vi "MGI CheckValue Directory Compare.vi"(5 "U32 Slider Ref (Use Progress Bar Dialog)":refnum<vi>, 7 "CheckValue Type (Checksum)":T1, 8 "error in (no error)":errorcluster, 9 "Expected CheckValue U32[i]":u32[](array[numeric]) format="%.0x", 10 "Relative Path[i]":path[](array[path]), 11 "Path":path) -> (0 "error out":errorcluster, 1 "Missing?[i]":bool[](array[boolean]), 2 "Missmatch or Missing?[i]":bool[](array[boolean]), 3 "All Match?":bool, 4 "Aborted?":bool, 6 "Actual CheckValue U32[i]":u32[](array[numeric]) format="%.0x")   [LabVIEW 2020]
doc: "Compare the specified expected files and checkvalues to the specified directory. Extra files in the directory are ignored. If all expected files match, then output true, otherwise output false.\nIf a reference to a slider is wired, then the slider is updated to show the progress of the comparison. Otherwise show a progress bar dialog with optional abort button.\n\nAuthored by Shawn Walpole\nsupport@mooregoodideas.com\nwww.mooregoodideas.com\n\nCopyright (c) 2010, Moore Good Ideas, Inc.\n\nAll rights reserved.\n\nRedistribution and use in source and binary forms, with or without modification, are permitted provided that the following conditions are met:\n\n * Redistributions of source code must retain the above copyright notice, this list of conditions and the following disclaimer.\n * Redistributions in binary form must reproduce the above copyright notice, this list of conditions and the following disclaimer in the documentation and/or other materials provided with the distribution.\n * Neither the name of Moore Good Ideas, Inc. nor the names of its contributors may be used to endorse or promote products derived from this software without specific prior written permission.\n\nTHIS SOFTWARE IS PROVIDED BY THE COPYRIGHT HOLDERS AND CONTRIBUTORS \"AS IS\" AND ANY EXPRESS OR IMPLIED WARRANTIES, INCLUDING, BUT NOT LIMITED TO, THE IMPLIED WARRANTIES OF MERCHANTABILITY AND FITNESS FOR A PARTICULAR PURPOSE ARE DISCLAIMED. IN NO EVENT SHALL THE COPYRIGHT OWNER OR CONTRIBUTORS BE LIABLE FOR ANY DIRECT, INDIRECT, INCIDENTAL, SPECIAL, EXEMPLARY, OR CONSEQUENTIAL DAMAGES (INCLUDING, BUT NOT LIMITED TO, PROCUREMENT OF SUBSTITUTE GOODS OR SERVICES; LOSS OF USE, DATA, OR PROFITS; OR BUSINESS INTERRUPTION) HOWEVER CAUSED AND ON ANY THEORY OF LIABILITY, WHETHER IN CONTRACT, STRICT LIABILITY, OR TORT (INCLUDING NEGLIGENCE OR OTHERWISE) ARISING IN ANY WAY OUT OF THE USE OF THIS SOFTWARE, EVEN IF ADVISED OF THE POSSIBILITY OF SUCH DAMAGE."
uses:
  <userlib>/_MGI/File/Checksum/MGI CheckValue Method Enum.ctl
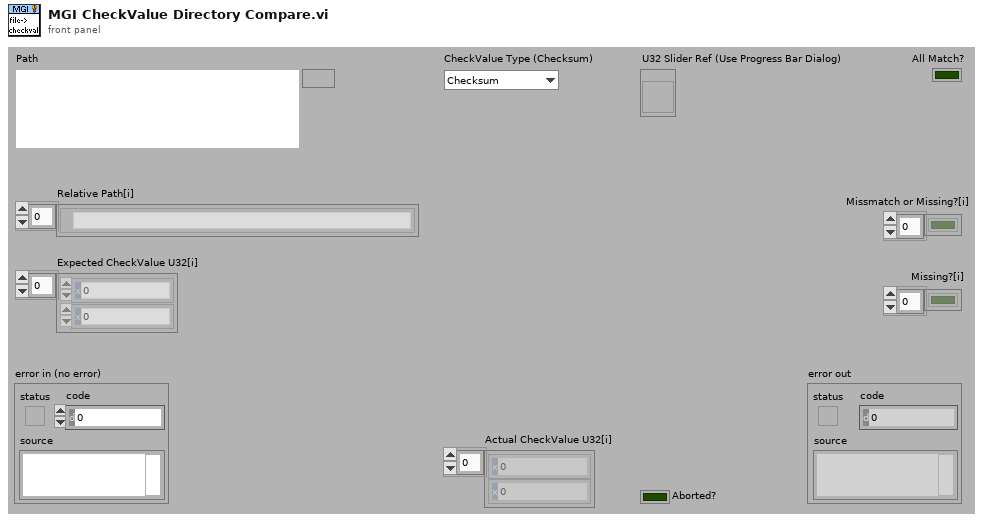
[diagram p1: front panel]
types:
  T1 = typedef "MGI CheckValue Method Enum.ctl" = enum16{"Checksum", "XOr"}
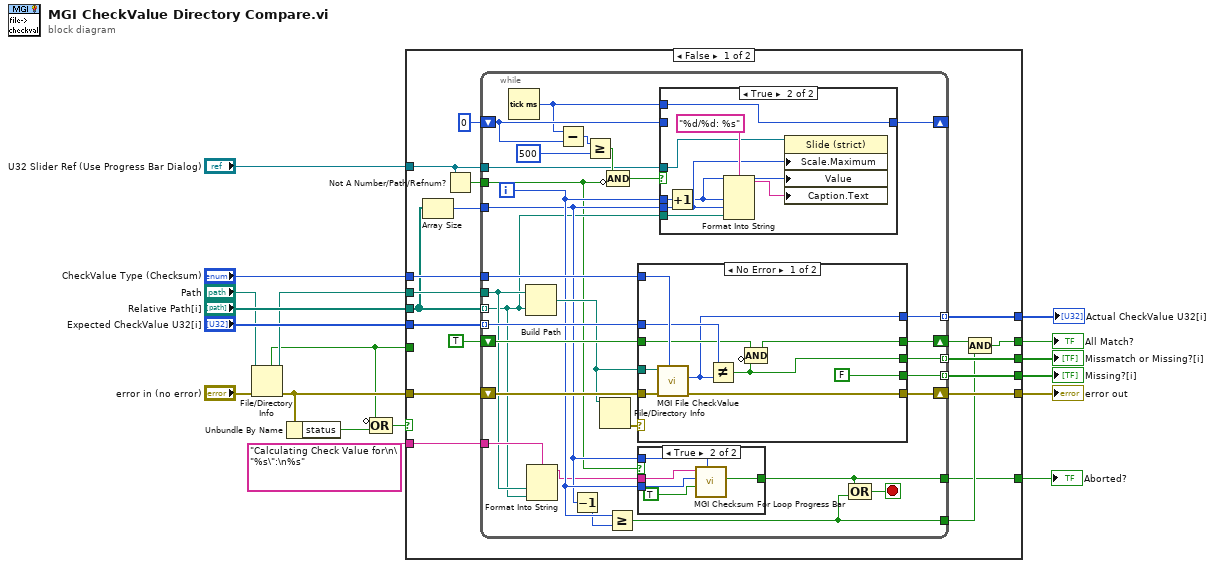
[diagram p0: block diagram]
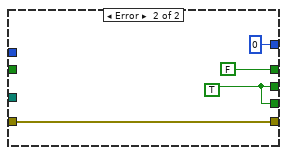
[diagram p4: hidden frame]
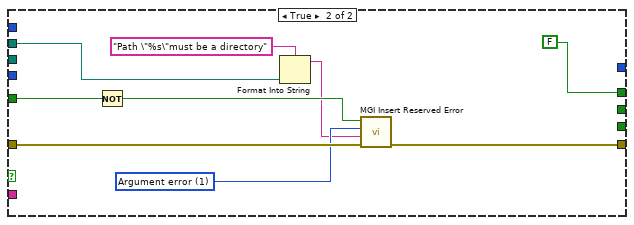
[diagram p5: hidden frame]
diagram:
  n1 = File/Directory Info(path="Path", error in="error in (no error)") -> (path out=w12:path, directory=w7:bool, error out=w9:errorcluster)  [unwired: 4 out]
  n2 = Unbundle By Name(w9) -> ("status"=w11:bool)
  n3 = Compound Arithmetic op=OR(invert w7, w11) -> (w10:bool)
  n4 = case shown="False" w10 {
    tunnel: "Relative Path[i]" -> [w24 _]
    tunnel: "Expected CheckValue U32[i]" -> [w37 _]
    tunnel: "CheckValue Type (Checksum)" -> [w36 _]
    tunnel: [w25 FALSE] -> w15
    tunnel: w12 -> [w34 w98]
    tunnel: w9 -> [w33 w104]
    tunnel: [w32 w103] -> w8
    tunnel: w7 -> [_ w101]
    tunnel: [w31 _] -> w6
    tunnel: [w30 _] -> w5
    tunnel: "U32 Slider Ref (Use Progress Bar Dialog)" -> [w27 _]
    tunnel: "Calculating Check Value for\n\"%s\":\n%s" ("format string") -> [w21 _]
    tunnel: [w20 _] -> w2
    tunnel: [w19 _] -> w1
    frame False {
      n5 = Array Size(array=w24) -> (size(s)=w23:i32)
      n6 = Not A Number/Path/Refnum?(number/path/refnum=w27) -> (NaN/Path/Refnum?=w29:bool)
      n7 = while {
        tunnel: w24 -> [w44] mode=indexing
        tunnel: w37 -> [w65] mode=indexing
        tunnel: w34 -> [w45]
        shift-right: [w58] -> w32
        shift-left: w33 -> [w67]
        tunnel: w36 -> [w66]
        shift-right: [w63] -> w26
        shift-left: TRUE -> [w64]
        tunnel: [w62] -> w31 mode=indexing
        tunnel: [w59] -> w30 mode=indexing
        shift-right: [w51] -> _
        shift-left: u32 0 ("millisecond timer value") -> [w52]
        tunnel: w27 -> [w53]
        tunnel: w29 -> [w40]
        tunnel: w23 -> [w48]
        tunnel: [w42] -> w22
        tunnel: w21 -> [w46]
        tunnel: [w39] -> w20
        tunnel: [w38] -> w19 mode=indexing
        i -> [w49]
        stop <- w41 stop-if-true
        n8 = Tick Count (ms)() -> (millisecond timer value=w50:u32)
        n9 = Build Path(base path=w45, name or relative path=w44) -> (appended path=w61:path)
        n10 = Format Into String(format string=w46, w45, w44) -> (resulting string=w43:string)  [unwired: 2 in, 1 out]
        n11 = Subtract(x=w50, y=w52) -> (x-y=w57:u32)
        n12 = Decrement(x=w48) -> (x-1=w47:i32)
        n13 = Greater Or Equal?(x=w57, y=u32 500) -> (x >= y?=w56:bool)
        n14 = File/Directory Info(path=w61) -> (error out=w60:errorcluster)  [unwired: 1 in, 6 out]
        n15 = Compound Arithmetic op=AND(w56, invert w40) -> (w54:bool)
        n16 = Greater Or Equal?(x=w49, y=w47) -> (x >= y?=w42:bool)
        n17 = case shown="No Error" w60 {
          tunnel: w67 -> [w91 w95]
          tunnel: w66 -> [w90 _]
          tunnel: w65 -> [w89 _]
          tunnel: w64 -> [w88 _]
          tunnel: [w87 FALSE] -> w63
          tunnel: [w84 w94] -> w62
          tunnel: w61 -> [w86 _]
          tunnel: [FALSE w94] -> w59
          tunnel: [w83 w95] -> w58
          tunnel: [w82 u32 0 ("CheckValue")] -> w38
          frame No Error {
            n18 = call <userlib>:"MGI File CheckValue.vi"("CheckValue Type"=w90, "error in (no error)"=w91, "File"=w86) -> ("error out"=w83:errorcluster, "CheckSum"=w82:u32)  [unwired: 7 in]
            n19 = Not Equal?(x=w89, y=w82) -> (x != y?=w84:bool)
            n20 = Compound Arithmetic op=AND(w88, invert w84) -> (w87:bool)
          }
          frame Error {
            w94 = TRUE
          }
        }
        n21 = case shown="True" w40 {
          tunnel: w49 -> [_ w70]
          tunnel: w48 -> [_ w68]
          tunnel: w43 -> [_ w71]
          tunnel: [_ w72] -> w39
          frame False {
          }
          frame True {
            n22 = call <userlib>:"MGI Checksum For Loop Progress Bar.vi"("Total Iter"=w68, "Allow Abort?(F)"=TRUE, "Current Iter"=w70, "Message"=w71) -> ("Aborted?"=w72:bool)  [unwired: 6 in, 1 out]
          }
        }
        n23 = case shown="True" w54 {
          tunnel: w53 -> [_ w78]
          tunnel: w49 -> [_ w75]
          tunnel: w48 -> [_ w79]
          tunnel: w52 -> [w73 _]
          tunnel: [w73 w77] -> w51
          tunnel: w50 -> [_ w77]
          tunnel: w44 -> [_ w76]
          frame False {
          }
          frame True {
            n24 = Increment(x=w75) -> (x+1=w74:i32)
            n25 = Format Into String(format string="%d/%d: %s", w74, w79, w76) -> (resulting string=w81:string)  [unwired: 2 in, 1 out]
            n26 = property class="Slide (strict)"(reference=w78, "Scale.Maximum"=w79, "Value"=w74, "Caption.Text"=w81) -> ()  [unwired: 1 in, 2 out]
          }
        }
        n27 = Compound Arithmetic op=OR(w39, w42) -> (w41:bool)
      }
      n28 = Compound Arithmetic op=AND(w26, w22) -> (w25:bool)
    }
    frame True {
      w99 = u16 1 items=["No error", "Argument error", "Memory is full", "Out of zone", "End of file", "File already open", "Generic file I/O error", "File not found", "File permission error", "Disk is full", "Duplicate path", "Too many files open", "System feature not enabled", "Resource file not found", "Cannot add resource", "Resource not found", "Image not found", "Image memory error", "Pen does not exist", "Config type invalid", "Config token not found", "Config parse error", "Config memory error", "Bad external code format", "Bad external code offset", "External code not present", "Null window", "Destroy window error", "Null menu", "Print aborted", "Bad print record", "Print driver error", "Windows error during printing", "Memory error during printing", "Print dialog error", "Generic print error", "Invalid device refnum", "Device not found", "Device parameter error", "Device unit error", "Cannot open device", "Device call aborted", "Generic error", "Cancelled by user", "Object ID too low", "Object ID too high", "Object not in heap", "Unknown heap", "Unknown object (invalid DefProc)", "Unknown object (DefProc not in table)", "Message out of range", "Invalid (null) method", "Unknown message", "Manager call not supported", "Bad address", "Network operation in progress", "Network operation timed out", "Connection is busy", "Network attribute not supported", "Network error", "Address in use", "System out of memory", "Connection aborted", "Connection refused", "Not connected", "Already connected", "Connection closed", "Initialization error (interapplication manager)", "Bad occurrence", "Wait on unbound occurrence handler", "Occurrence queue overflow", "Datalog type conflict", "Unused", "Unrecognized type (interapplication manager)", "Memory corrupt", "Failed to make temporary DLL", "Old CIN version", "Drag socket not found", "Failed to load drop-object", "Failed to register OLE object", "Failed to release OLE object", "Format specifier type mismatch", "Unknown format specifier", "Too few format specifiers", "Too many format specifiers", "Scan failed", "Newer CIN version", "OLE Convert", "Runtime menu error", "Password tampered", "Unknown error code"] ("Reserved Error Code (Generic error)")
      n29 = Not(x=w101) -> (.not. x?=w100:bool)
      n30 = Format Into String(format string="Path \"%s\"must be a directory", w98) -> (resulting string=w97:string)  [unwired: 2 in, 1 out]
      n31 = call <userlib>:"MGI Insert Reserved Error.vi"("Error In"=w104, "Error Description"=w97, "Reserved Error Code (Generic error)"=w99, "Error? (T)"=w100) -> ("Error Out"=w103:errorcluster)  [unwired: 7 in]
    }
  }
  "error out" <- w8
  "All Match?" <- w15
  "Missmatch or Missing?[i]" <- w6
  "Missing?[i]" <- w5
  "Aborted?" <- w2
  "Actual CheckValue U32[i]" <- w1
